vi "login.vi"() -> (0 "error out":errorcluster, 3 "Device Out":T1)   [LabVIEW 2019]
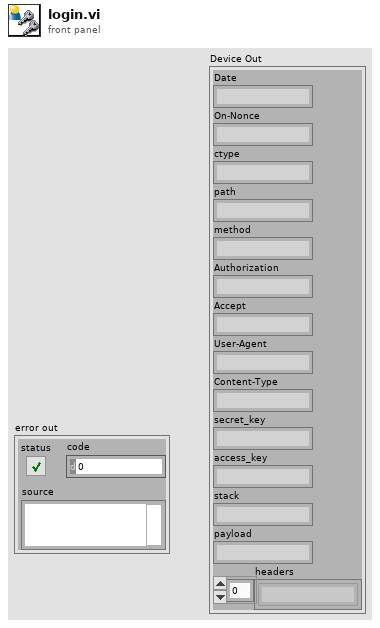
[diagram p1: front panel]
types:
  T1 = cluster{"Date":string, "On-Nonce":string, "ctype":string, "path":string, "method":string, "Authorization":string, "Accept":string, "User-Agent":string, "Content-Type":string, "secret_key":string, "access_key":string, "stack":string, "payload":string, "headers":string[]}
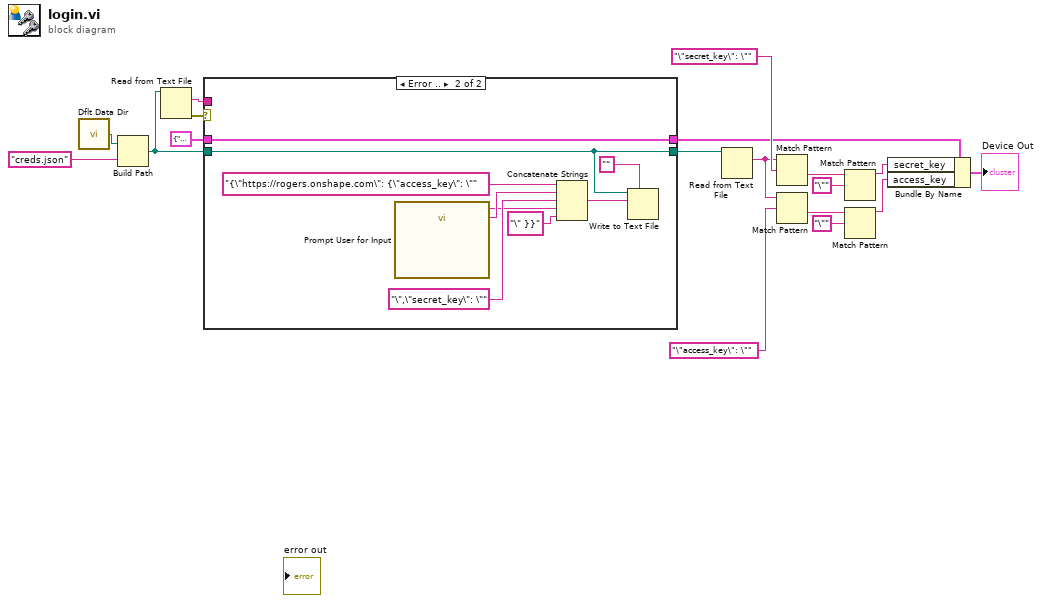
[diagram p0: block diagram]
diagram:
  n1 = call <vilib>:"Dflt Data Dir.vi"() -> ("App:Default Data Directory"=w5:path)
  n2 = Build Path(base path=w5, name or relative path="creds.json") -> (appended path=w3:path)
  n3 = Read from Text File(file (use dialog)=w3) -> (text=w16:string, error out=w18:errorcluster)  [unwired: 3 in, 2 out]
  n4 = case shown="Error .." w18 {
    tunnel: T1 {"Date"="", "On-Nonce"="", "ctype"="", "path"="", "method"="", "Authorization"="", "Accept"="", "User-Agent"="", "Content-Type"="", "secret_key"="", "access_key"="", "stack"="", "payload"="", "headers"=[]} ("Device In") -> [w20 w23]
    tunnel: w16 -> [_ _]
    tunnel: w3 -> [w19 w21]
    tunnel: [w20 w23] -> w7
    tunnel: [w19 w21] -> w2
    frame No Error {
    }
    frame Error {
      n5 = call "Prompt User for Input"() -> ("secret_key"=w26:string, "access_key"=w28:string)  [unwired: 16 in, 2 out]
      n6 = Concatenate Strings("{\"https://rogers.onshape.com\": {\"access_key\": \"", w28, "\",\"secret_key\": \"", w26, "\" }}") -> (w24:string)
      n7 = Write to Text File(prompt (Choose or enter file path)="", file (use dialog)=w21, text=w24) -> ()  [unwired: 1 in, 3 out]
    }
  }
  n8 = Read from Text File(file (use dialog)=w2) -> (text=w6:string)  [unwired: 3 in, 3 out]
  n9 = Match Pattern(string=w6, regular expression="\"secret_key\": \"") -> (after substring=w12:string)  [unwired: 1 in, 3 out]
  n10 = Match Pattern(string=w6, regular expression="\"access_key\": \"") -> (after substring=w13:string)  [unwired: 1 in, 3 out]
  n11 = Match Pattern(string=w12, regular expression="\"") -> (before substring=w14:string)  [unwired: 1 in, 3 out]
  n12 = Match Pattern(string=w13, regular expression="\"") -> (before substring=w15:string)  [unwired: 1 in, 3 out]
  n13 = Bundle By Name(cluster=w7, "secret_key"=w14, "access_key"=w15) -> (→"Device Out":T1)
